vi "test generate sample array.vi"() -> ()   [LabVIEW 2018, in "LV-Julia_ZMQ-Roundtrip_lib.lvlib"]
uses:
  LV-Julia_ZMQ-Roundtrip_lib.lvlib
  e5e6068f-5182-42d9-b78c-40292424fa1f.vi
panel:
  out "Array 3D":csg[][][](array[numeric])
  out "Array 2D":csg[][](array[numeric])
  out "Array 1D":csg[](array[numeric])
  in  "type":csg
  in  "dims":u8=3 min=1 max=3
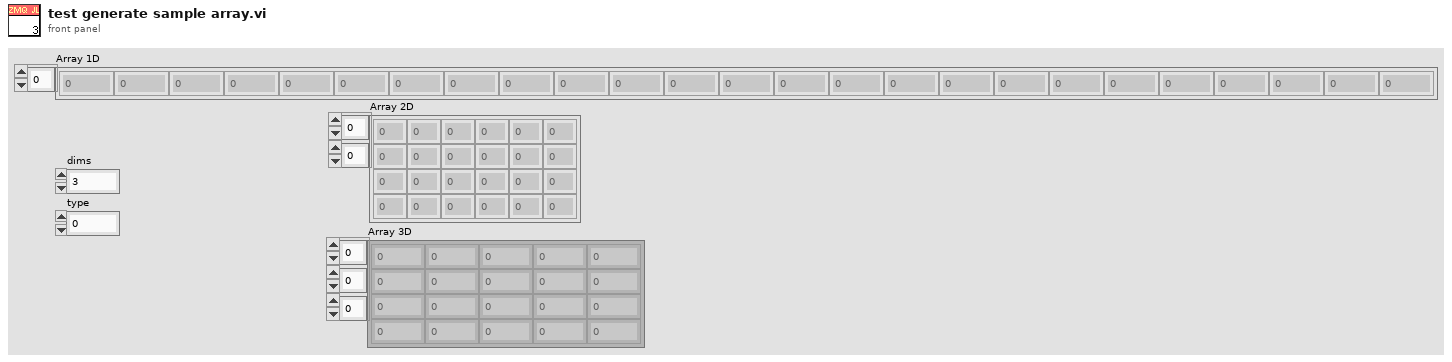
[diagram p1: front panel]
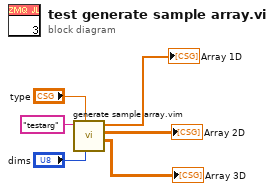
[diagram p0: block diagram]
diagram:
  n1 = call "generate sample array.vim"("Bindata & descr in"="dims", "type"="type", "kwarg_name"="testarg") -> ("Array 3D"=→"Array 3D":csg[][][], "Array 2D"=→"Array 2D":csg[][], "Array 1D"=→"Array 1D":csg[])  [unwired: 3 in, 3 out]
